vi "ELVIS III v1.0 Configure IO.vi"(7 "Value":bool, 8 "error in (no error)":errorcluster, 9 "Bitmask Array":bool[][](array[boolean]), 10 "Bitcode Array":bool[][](array[boolean]), 11 "myRIO FPGA Ref In":T1) -> (0 "error out":errorcluster)   [LabVIEW 2021]
uses:
  <vilib>/myRIO/Common/Instrument Driver Framework/Utilities/typedefs/Generic FPGA Reference.ctl
  <vilib>/myRIO/Common/Instrument Driver Framework/ELVIS III v1.0/Resource Manager/typedefs/ELVIS III IO Config FPGA Reference.ctl
  <vilib>/myRIO/Common/Instrument Driver Framework/ELVIS III v1.0/Resource Manager/typedefs/ELVIS III v1.0 Connector List.ctl
  <vilib>/Utility/error.llb/Error Cluster From Error Code.vi
  <vilib>/rvi/errors/niLvFpgaAdjustHostInterfaceError.vi
  <vilib>/rvi/interface/nirviReadWriteControl/nirviReadWriteControl.xnode
  NiFpgaLv.dll
  <vilib>/rvi/interface/Simulation/niFpgaSimulationCallBeginRW.vi
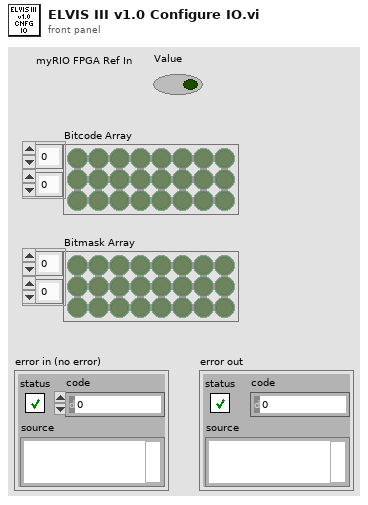
[diagram p1: front panel]
types:
  T1 = typedef "Generic FPGA Reference.ctl" = refnum<k20>
  T2 = typedef "ELVIS III IO Config FPGA Reference.ctl" = refnum<k20>
  T3 = typedef "ELVIS III v1.0 Connector List.ctl" = enum32{"None", "ConnectorA", "ConnectorB"}
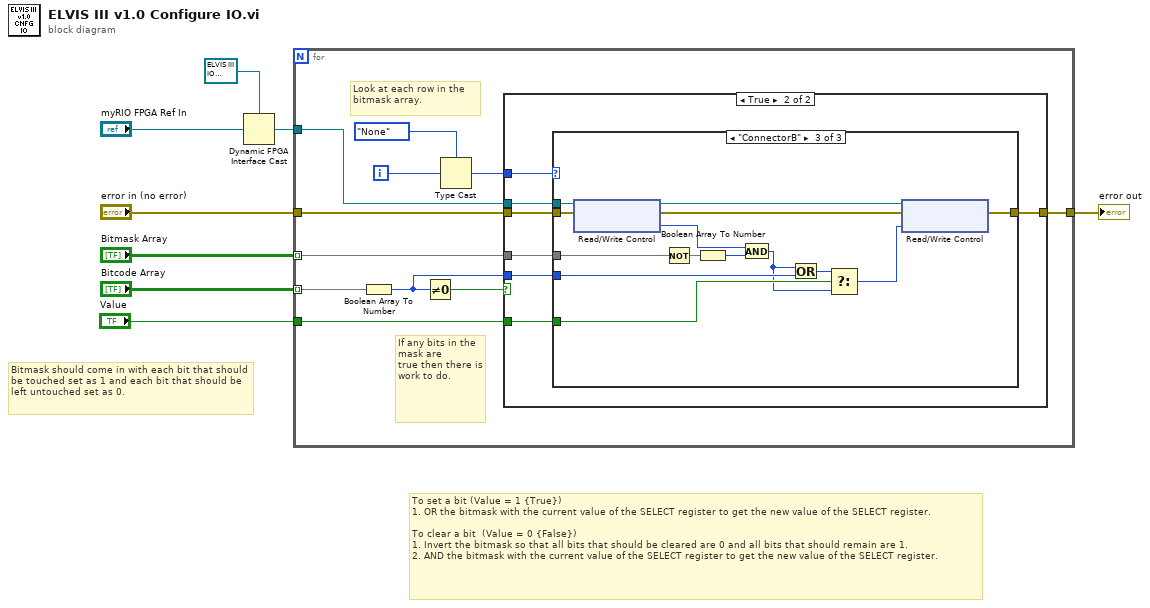
[diagram p0: block diagram]
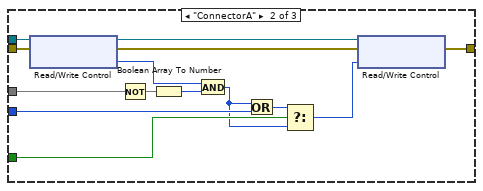
[diagram p4: hidden frame]
diagram:
  # "To set a bit (Value = 1 {True}) \n1. OR the bitmask with the current value of the SELECT register to get the new value of the SELECT register.\n\nTo clear a bit  (Value = 0 {False})\n1. Invert the bitmask so that all bits that should be cleared are 0 and all bits that should remain are 1.\n2. AND the bitmask with the current value of the SELECT register to get the new value of the SELECT register."
  # "Bitmask should come in with each bit that should be touched set as 1 and each bit that should be left untouched set as 0."
  n1 = Dynamic FPGA Interface Cast(Session In=T2 refnum ("FPGA Interface"), Type="myRIO FPGA Ref In") -> (Session Out=w4:T2)
  n2 = for {
    tunnel: w4 -> [w19]
    tunnel: "error in (no error)" -> [w18]
    tunnel: [w17] -> w7
    tunnel: "Bitcode Array" -> [w10] mode=indexing
    tunnel: "Value" -> [w13]
    tunnel: "Bitmask Array" -> [w9] mode=indexing
    i -> [w16]
    # "If any bits in the mask are\ntrue then there is work to do."
    # "Look at each row in the bitmask array."
    n3 = Boolean Array To Number(Boolean array=w10) -> (number=w11:u64)
    n4 = Not Equal To 0?(x=w11) -> (x != 0?=w12:bool)
    n5 = Type Cast(type=ELVIS_III_v1.0_Connector_List."None" ("Connector List"), x=w16) -> (*(type *) &x=w15:T3)
    n6 = case shown="True" w12 {
      tunnel: w19 -> [_ w27]
      tunnel: w18 -> [w20 w26]
      tunnel: [w20 w25] -> w17
      tunnel: w15 -> [_ w24]
      tunnel: w13 -> [_ w23]
      tunnel: w11 -> [_ w22]
      tunnel: w9 -> [_ w21]
      frame False {
        # "There are no bits to change for this connector."
      }
      frame True {
        n7 = case shown="\"ConnectorB\"" w24 {
          tunnel: w27 -> [_ w41 w55]
          tunnel: w26 -> [w28 w42 w56]
          tunnel: [w28 w40 w54] -> w25
          tunnel: w23 -> [_ w33 w47]
          tunnel: w22 -> [_ w34 w48]
          tunnel: w21 -> [_ w29 w43]
          frame "None", Default {
            # "Do Nothing"
          }
          frame "ConnectorA" {
            n8 = xnode "Read/Write Control"("FPGA VI Reference In"=w41, "error in"=w42) -> ("FPGA VI Reference Out"=w38:T2, "error out"=w39:errorcluster, "SYS.SELECTA"=w37:u64)
            n9 = Not(x=w29) -> (.not. x?=w36:bool[])
            n10 = Boolean Array To Number(Boolean array=w36) -> (number=w35:u64)
            n11 = And(x=w37, y=w35) -> (x .and. y?=w32:u64)
            n12 = Or(x=w32, y=w34) -> (x .or. y?=w31:u64)
            n13 = Select(t=w31, s=w33, f=w32) -> (s? t:f=w30:u64)
            n14 = xnode "Read/Write Control"("FPGA VI Reference In"=w38, "error in"=w39, "SYS.SELECTA"=w30) -> ("error out"=w40:errorcluster)  [unwired: 1 out]
          }
          frame "ConnectorB" {
            n15 = xnode "Read/Write Control"("FPGA VI Reference In"=w55, "error in"=w56) -> ("FPGA VI Reference Out"=w52:T2, "error out"=w53:errorcluster, "SYS.SELECTB"=w51:u64)
            n16 = Not(x=w43) -> (.not. x?=w50:bool[])
            n17 = Boolean Array To Number(Boolean array=w50) -> (number=w49:u64)
            n18 = And(x=w51, y=w49) -> (x .and. y?=w46:u64)
            n19 = Or(x=w46, y=w48) -> (x .or. y?=w45:u64)
            n20 = Select(t=w45, s=w47, f=w46) -> (s? t:f=w44:u64)
            n21 = xnode "Read/Write Control"("FPGA VI Reference In"=w52, "error in"=w53, "SYS.SELECTB"=w44) -> ("error out"=w54:errorcluster)  [unwired: 1 out]
          }
        }
      }
    }
  }
  "error out" <- w7
